vi "VerifyComputer.vi"(10 "verification file path":path) -> (2 "OK?":bool)   [LabVIEW 2019, in "Tools.lvlib"]
uses:
  Tools.lvlib
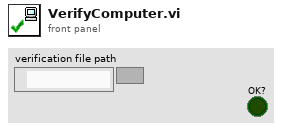
[diagram p1: front panel]
types:
  T1 = enum16{"open", "replace", "create", "open or create", "replace or create", "replace or create with confirmation"}
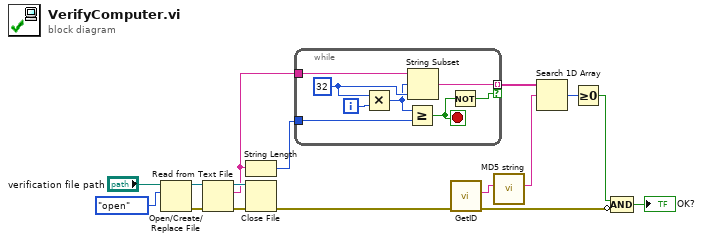
[diagram p0: block diagram]
diagram:
  n1 = Open/Create/Replace File(file path (use dialog)="verification file path", operation (0:open)=T1."open") -> (refnum out=w12:refnum<file>, error out=w13:errorcluster)  [unwired: 4 in, 1 out]
  n2 = Read from Text File(file (use dialog)=w12, error in=w13) -> (refnum out=w11:refnum<file>, text=w9:string, error out=w10:errorcluster)  [unwired: 2 in, 1 out]
  n3 = String Length(string=w9) -> (length=w15:i32)
  n4 = Close File(refnum=w11, error in=w10) -> (error out=w6:errorcluster)  [unwired: 1 out]
  n5 = while {
    tunnel: w9 -> [w24]
    tunnel: [w21] -> w8 mode=indexing if=w17
    tunnel: w15 -> [w19]
    i -> [w23]
    stop <- w18 stop-if-true
    w22 = 32 ("x")
    n6 = Multiply(x=w22, y=w23) -> (x*y=w20:i32)
    n7 = Greater Or Equal?(x=w20, y=w19) -> (x >= y?=w18:bool)
    n8 = String Subset(string=w24, offset (0)=w20, length (rest)=w22) -> (substring=w21:string)
    n9 = Not(x=w18) -> (.not. x?=w17:bool)
  }
  n10 = call "GetID.vi"("error in (no error)"=w6) -> ("error out"=w4:errorcluster, "Computer ID"=w1:string)  [unwired: 9 in]
  n11 = call "MD5 string.vi"("Message String"=w1) -> ("MD5 message-digest"=w7:string)  [unwired: 10 in]
  n12 = Search 1D Array(1D array=w8, element=w7) -> (index of element=w16:i32)  [unwired: 1 in]
  n13 = Greater Or Equal To 0?(x=w16) -> (x >= 0?=w5:bool)
  n14 = Compound Arithmetic op=AND(w5, invert w4) -> (→"OK?":bool)
